vi "Test Report Error Codes.vi"(8 "error in (no error)":errorcluster) -> (0 "error out":errorcluster)   [LabVIEW 2020]
uses:
  <vilib>/Utility/sysdir.llb/System Directory Type.ctl
  classes/Test Report.Default/Test Report.Default.lvclass
  classes/Assert/Assert Equal Value_Variant.vi
  classes/Test/Test.lvclass
  classes/Assert/Assert.lvclass
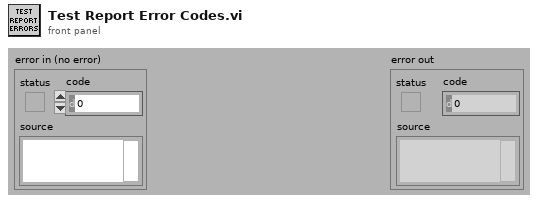
[diagram p1: front panel]
types:
  T1 = typedef "System Directory Type.ctl" = i32
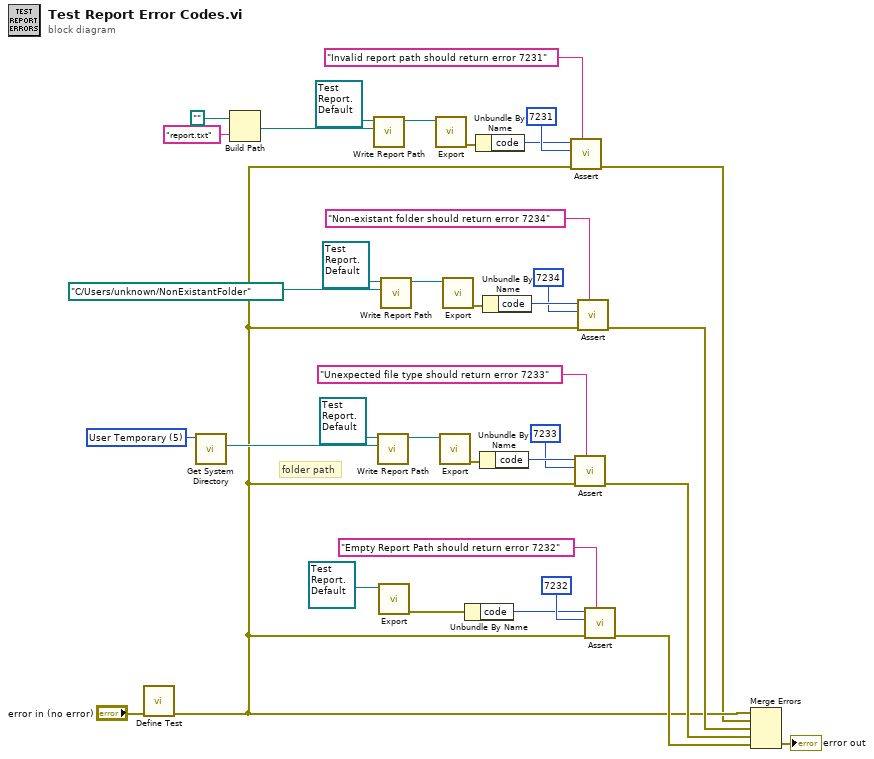
[diagram p0: block diagram]
diagram:
  w29 = T1 5 items=["User Home"=0, "User Desktop"=1, "User Documents"=2, "User Application Data"=3, "User Preferences"=4, "User Temporary"=5, "Public Documents"=6, "Public Application Data"=7, "Public Preferences"=8, "Public Cache"=13, "System Core Libraries"=9, "System Installed Libraries"=10, "Application Files"=11, "Boot Volume Root"=12] ("system directory type")
  # "folder path"
  n1 = call "Define Test.vi"("error in (no error)"="error in (no error)") -> ("error out"=w14:errorcluster)  [unwired: 9 in, 1 out]
  n2 = call <vilib>:"Get System Directory.vi"("system directory type"=w29) -> ("system directory"=w28:path)  [unwired: 10 in]
  n3 = Build Path(base path=path "", name or relative path="report.txt") -> (appended path=w20:path)
  n4 = call "Write Report Path.vi"("Report Path"=w20, "Test Report.Default in"=refnum<class "Test Report.Default.lvclass"> refnum ("Caraya.lvlib:Test Report.Default.lvclass")) -> ("Test Report.Default out"=w22:refnum<class "Test Report.Default.lvclass">)  [unwired: 9 in]
  n5 = call "Write Report Path.vi"("Report Path"=w28, "Test Report.Default in"=refnum<class "Test Report.Default.lvclass"> refnum ("Caraya.lvlib:Test Report.Default.lvclass")) -> ("Test Report.Default out"=w31:refnum<class "Test Report.Default.lvclass">)  [unwired: 9 in]
  n6 = call-dynamic "Export.vi"("Test Report in"=refnum<class "Test Report.Default.lvclass"> refnum ("Caraya.lvlib:Test Report.Default.lvclass")) -> ("error out"=w33:errorcluster)  [unwired: 9 in, 1 out]
  n7 = call "Write Report Path.vi"("Report Path"=path "C:/Users/unknown/NonExistantFolder", "Test Report.Default in"=refnum<class "Test Report.Default.lvclass"> refnum ("Caraya.lvlib:Test Report.Default.lvclass")) -> ("Test Report.Default out"=w26:refnum<class "Test Report.Default.lvclass">)  [unwired: 9 in]
  n8 = call-dynamic "Export.vi"("Test Report in"=w22) -> ("error out"=w21:errorcluster)  [unwired: 9 in, 1 out]
  n9 = call-dynamic "Export.vi"("Test Report in"=w31) -> ("error out"=w30:errorcluster)  [unwired: 9 in, 1 out]
  n10 = call-dynamic "Export.vi"("Test Report in"=w26) -> ("error out"=w27:errorcluster)  [unwired: 9 in, 1 out]
  n11 = Unbundle By Name(w33) -> ("code"=w1:i32)
  n12 = Unbundle By Name(w21) -> ("code"=w11:i32)
  n13 = Unbundle By Name(w30) -> ("code"=w5:i32)
  n14 = Unbundle By Name(w27) -> ("code"=w8:i32)
  n15 = call-poly "Assert.vi"("Label"="Invalid report path should return error 7231", "error in (no error)"=w14, "Y"=7231 ("code"), "X"=w11) -> ("error out"=w13:errorcluster)  [unwired: 6 in, 1 out]
  n16 = call-poly "Assert.vi"("Label"="Unexpected file type should return error 7233", "error in (no error)"=w14, "Y"=7233 ("code"), "X"=w5) -> ("error out"=w16:errorcluster)  [unwired: 6 in, 1 out]
  n17 = call-poly "Assert.vi"("Label"="Non-existant folder should return error 7234", "error in (no error)"=w14, "Y"=7234 ("code"), "X"=w8) -> ("error out"=w15:errorcluster)  [unwired: 6 in, 1 out]
  n18 = call-poly "Assert.vi"("Label"="Empty Report Path should return error 7232", "error in (no error)"=w14, "Y"=7232 ("code"), "X"=w1) -> ("error out"=w17:errorcluster)  [unwired: 6 in, 1 out]
  n19 = Merge Errors(w14, w13, w15, w16, w17) -> (→"error out":errorcluster)
